vi "resonant.z.stack.run_rrMD.vi"() -> ()   [LabVIEW 2012]
doc: "SciScan 1.2 160622"
uses:
  Custom Controls/experiment type.ctl
  <vilib>/Utility/VariantDataType/Type.ctl
  GFG/GFGnumericGet.vi
  GFG/GFGfpRefGet.vi
  GFG/GFGbooleanGet.vi
  GFG/GFG library.lvlib
  <vilib>/Utility/VariantDataType/VariantType.lvlib
panel:
  out "error out 2":errorcluster
  out "transposed array":dbl[][](array[numeric])
  out "data":dbl[][](array[numeric])
  in  "error in (no error)":errorcluster
  out "error out":errorcluster
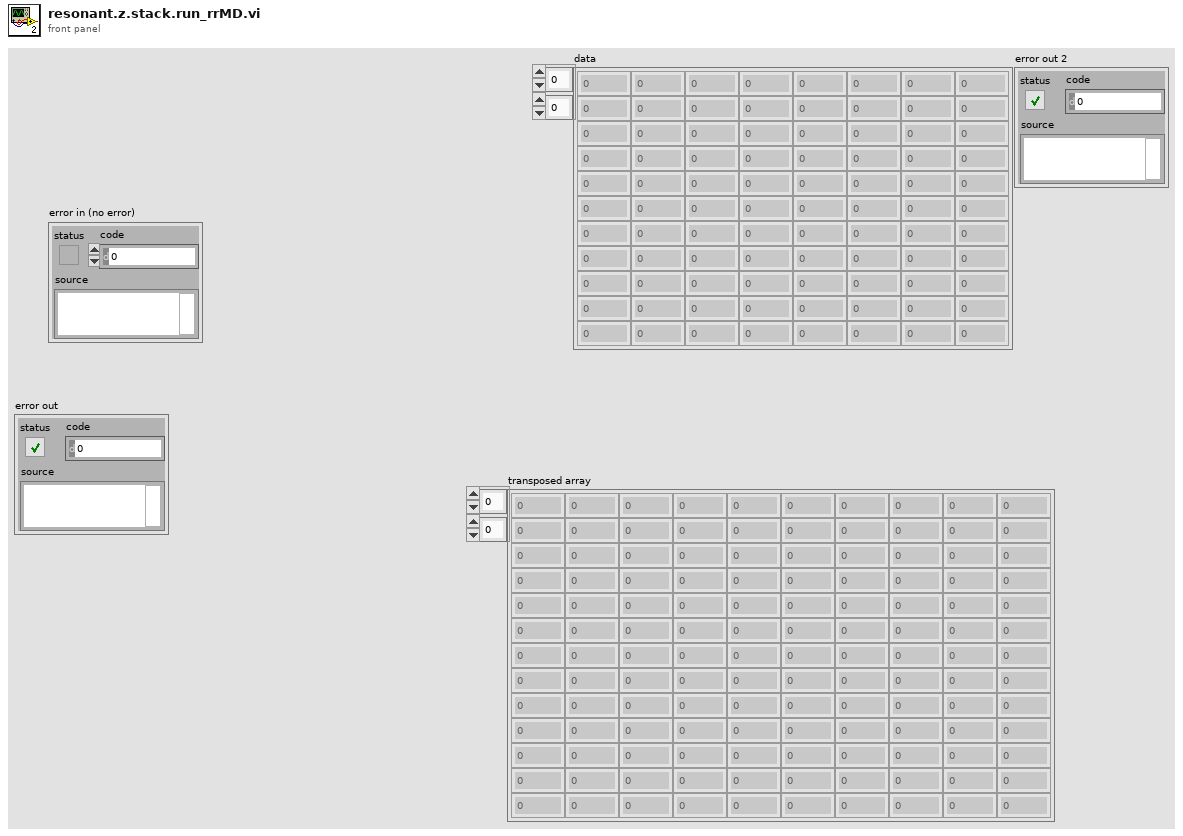
[diagram p1: front panel]
types:
  T1 = typedef "experiment type.ctl" = string
  T2 = enum8{"Enabled", "Disabled", "Disabled and Grayed Out"}
  T3 = cluster{"moveXabs":dbl, "moveYabs":dbl, "moveZabs":dbl}
  T4 = cluster{"WaveformChartRef":refnum<vi>, "DigitalRef":refnum<vi>, "ArrayRef":refnum<vi>, "TabControlRef":refnum<vi>, "EnumRef":refnum<vi>, "RingRef":refnum<vi>, "BooleanRef":refnum<vi>, "KnobRef":refnum<vi>, "SlideRef":refnum<vi>, "PathRef":refnum<vi>, "StringRef":refnum<vi>, "ComboBox":refnum<vi>, "WaveformGraphRef":refnum<vi>}
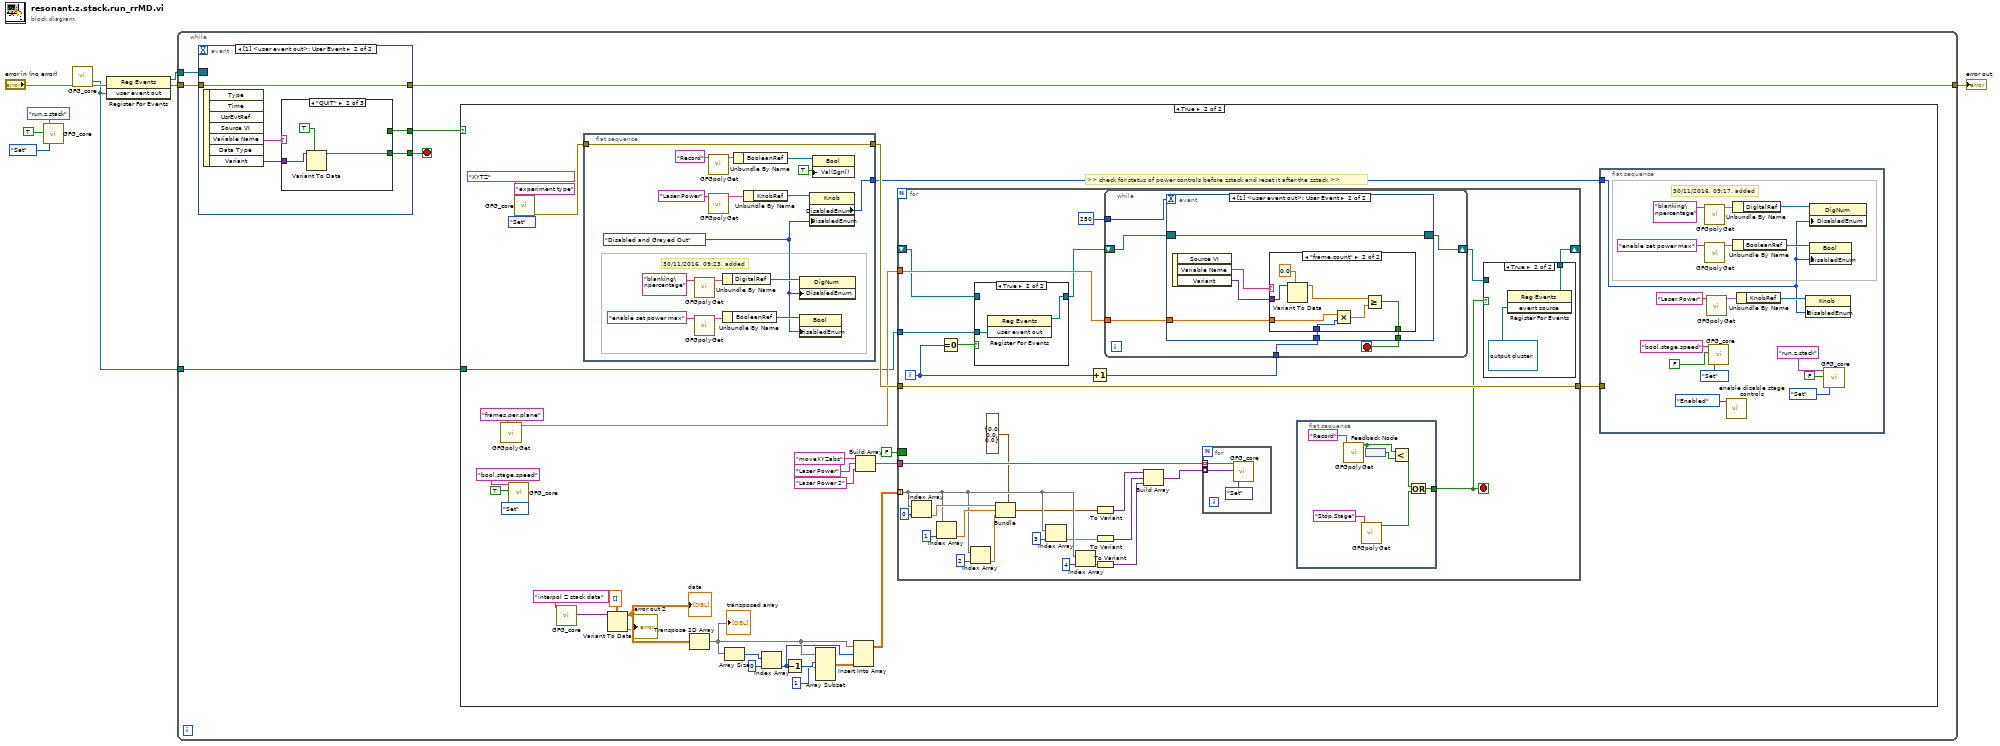
[diagram p0: block diagram]
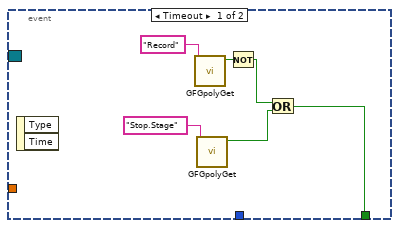
[diagram p5: hidden frame]
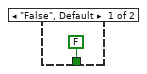
[diagram p6: hidden frame]
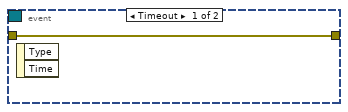
[diagram p7: hidden frame]
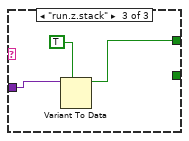
[diagram p9: hidden frame]
diagram:
  n1 = call "GFG_core.vi"("Variable Name in"="run.z.stack", "Variant in"=TRUE, "Action"=enum16{"Init", "Set", "Get"}."Set") -> ()  [unwired: 10 in, 7 out]
  n2 = call "GFG_core.vi"("error in (no error)"="error in (no error)") -> ("user event out"=w1:refnum<user-event>, "error out"=w6:errorcluster)  [unwired: 12 in, 5 out]
  n3 = register-events(error in=w6, w1) -> (reference out=w5:refnum<event-registration>, error out=w8:errorcluster)  [unwired: 1 in]
  n4 = while {
    tunnel: w5 -> [w15]
    tunnel: w8 -> [w14]
    tunnel: [w13] -> w9
    tunnel: w1 -> [w10]
    stop <- w12 stop-if-true
    n5 = event shown="[1] <user event out>: User Event" {
      selector: w15 -> [_ _]
      dyn-events: _ -> [_ _]
      timeout: _ -> [_ _]
      tunnel: w14 -> [w152 w157]
      tunnel: [w152 w157] -> w13
      tunnel: [_ w154] -> w12
      tunnel: [_ w153] -> w11
      event Timeout {
        n6 = event-data() -> ()  [unwired: 1 in, 2 out]
      }
      event User Event {
        n7 = event-data() -> ("Variable Name"=w156:string, "Variant"=w155:variant)  [unwired: 1 in, 5 out]
        n8 = case shown="\"QUIT\"" w156 {
          tunnel: w155 -> [_ w159 w162]
          tunnel: [_ w158 _] -> w154
          tunnel: [_ _ w161] -> w153
          frame "False", Default {
          }
          frame "QUIT" {
            n9 = Variant To Data(type=TRUE, Variant=w159) -> (data=w158:bool)  [unwired: 1 in, 1 out]
          }
          frame "run.z.stack" {
            n10 = Variant To Data(type=TRUE, Variant=w162) -> (data=w161:bool)  [unwired: 1 in, 1 out]
          }
        }
      }
    }
    n11 = case shown="True" w11 {
      tunnel: w10 -> [_ w17]
      frame False {
      }
      frame True {
        # ">> check for status of power controls before zstack and reset it after the zstack >>"
        n12 = call-poly "GFGpolyGet.vi"("Variable Name in"="frames.per.plane") -> ("Numeric"=w30:dbl)  [unwired: 8 in, 2 out]
        n13 = call "GFG_core.vi"("Variable Name in"="bool.stage.speed", "Variant in"=TRUE, "Action"=enum16{"Init", "Set", "Get"}."Set") -> ()  [unwired: 10 in, 7 out]
        n14 = call "GFG_core.vi"("Variable Name in"="experiment type", "Variant in"=T1 "XYTZ" ("experiment type"), "Action"=enum16{"Init", "Set", "Get"}."Set") -> ("error out"=w32:errorcluster)  [unwired: 10 in, 6 out]
        n15 = call "GFG_core.vi"("Variable Name in"="interpol Z stack data") -> ("Variant Out"=w44:variant)  [unwired: 12 in, 6 out]
        n16 = flat-sequence {
          tunnel: [w61] -> w33
          tunnel: w32 -> [w61]
          tunnel: [w47] -> w16
          frame #0 {
            w48 = T2."Disabled and Grayed Out" ("Disabled")
            # "30/11/2016, 09:23, added"
            n17 = call-poly "GFGpolyGet.vi"("Variable Name in"="blanking\npercentage") -> ("output cluster"=w53:T4)  [unwired: 9 in, 1 out]
            n18 = call-poly "GFGpolyGet.vi"("Variable Name in"="enable set power max") -> ("output cluster"=w50:T4)  [unwired: 9 in, 1 out]
            n19 = call-poly "GFGpolyGet.vi"("Variable Name in"="Record") -> ("output cluster"=w60:T4)  [unwired: 9 in, 1 out]
            n20 = call-poly "GFGpolyGet.vi"("Variable Name in"="Laser.Power") -> ("output cluster"=w55:T4)  [unwired: 9 in, 1 out]
            n21 = Unbundle By Name(w53) -> ("DigitalRef"=w54:refnum<vi>)
            n22 = Unbundle By Name(w50) -> ("BooleanRef"=w49:refnum<vi>)
            n23 = Unbundle By Name(w60) -> ("BooleanRef"=w59:refnum<vi>)
            n24 = Unbundle By Name(w55) -> ("KnobRef"=w57:refnum<vi>)
            n25 = property class="DigNum"(reference=w54, "DisabledEnum"=w48) -> ()  [unwired: 1 in, 2 out]
            n26 = property class="Bool"(reference=w49, "DisabledEnum"=w48) -> ()  [unwired: 1 in, 2 out]
            n27 = property class="Knob"(reference=w57, "DisabledEnum"=w48) -> ("DisabledEnum"=w47:T2)  [unwired: 1 in, 2 out]
            n28 = property class="Bool"(reference=w59, "Val(Sgnl)"=TRUE) -> ()  [unwired: 1 in, 2 out]
          }
        }
        n29 = Variant To Data(type=dbl[][] [] ("Interpolated Data"), Variant=w44) -> (data=w42:dbl[][], error out=→"error out 2":errorcluster)  [unwired: 1 in]
        "data" <- w42
        n30 = Transpose 2D Array(2D array=w42) -> (transposed array=w22:dbl[][])
        "transposed array" <- w22
        n31 = Array Size(array=w22) -> (size(s)=w26:i32[])
        n32 = Index Array(array=w26, index=0) -> (element=w20:i32)
        n33 = Decrement(x=w20) -> (x-1=w24:i32)
        n34 = Array Subset(array=w22, index (row)=w24, length (row)=1 ("length")) -> (w21:dbl[][])  [unwired: 2 in]
        n35 = Insert Into Array(array=w22, index (row)=w20, new element=w21) -> (w19:dbl[][])  [unwired: 1 in]
        n36 = Build Array("moveXYZabs" ("Variable Name in"), "Laser Power" ("Variable Name in"), "Laser Power 2" ("Variable Name in")) -> (w38:string[])
        n37 = for {
          tunnel: w19 -> [w100] mode=indexing
          tunnel: w38 -> [w109]
          tunnel: w33 -> [w90]
          tunnel: [w90] -> w34
          tunnel: w30 -> [w91]
          tunnel: w17 -> [w86]
          shift-right: [w82] -> _
          shift-left: _ -> [w84]
          border: FALSE ("Boolean Value OUT") -> [_]
          i -> [w88]
          stop <- w81 stop-if-true
          n38 = Index Array(array=w100, index=0) -> (element=w107:dbl)
          n39 = Index Array(array=w100, index=1) -> (element=w106:dbl)
          n40 = Equal To 0?(x=w88) -> (x = 0?=w87:bool)
          n41 = Index Array(array=w100, index=2) -> (element=w103:dbl)
          n42 = case shown="True" w87 {
            tunnel: w86 -> [_ w115]
            tunnel: [w113 w114] -> w85
            tunnel: w84 -> [w113 _]
            frame False {
            }
            frame True {
              n43 = register-events(w115) -> (reference out=w114:refnum<event-registration>)  [unwired: 2 in, 1 out]
            }
          }
          n44 = Bundle(cluster=T3 {"moveXabs"=0.0, "moveYabs"=0.0, "moveZabs"=0.0} ("output cluster"), "moveXabs"=w107, "moveYabs"=w106, "moveZabs"=w103) -> (w97:T3)
          n45 = Index Array(array=w100, index=3) -> (element=w98:dbl)
          n46 = Index Array(array=w100, index=4) -> (element=w99:dbl)
          n47 = Increment(x=w88) -> (x+1=w80:i32)
          n48 = To Variant(anything=w97) -> (Variant=w96:variant)
          n49 = To Variant(anything=w98) -> (Variant=w95:variant)
          n50 = To Variant(anything=w99) -> (Variant=w94:variant)
          n51 = while {
            tunnel: w91 -> [w120]
            tunnel: w80 -> [w119]
            tunnel: 250 -> [w117]
            shift-right: [w116] -> w83
            shift-left: w85 -> [w121]
            stop <- w118 stop-if-true
            n52 = event shown="[1] <user event out>: User Event" {
              selector: w121 -> [_ w128]
              dyn-events: [_ w128] -> w116
              timeout: w117 -> [_ _]
              tunnel: w120 -> [_ w131]
              tunnel: w119 -> [_ w130]
              tunnel: [w122 w129] -> w118
              event Timeout {
                n53 = event-data() -> ()  [unwired: 1 in, 2 out]
                n54 = call-poly "GFGpolyGet.vi"("Variable Name in"="Record") -> ("Boolean Value OUT"=w125:bool)  [unwired: 9 in, 1 out]
                n55 = call-poly "GFGpolyGet.vi"("Variable Name in"="Stop.Stage") -> ("Boolean Value OUT"=w126:bool)  [unwired: 9 in, 1 out]
                n56 = Not(x=w125) -> (.not. x?=w127:bool)
                n57 = Or(x=w127, y=w126) -> (x .or. y?=w122:bool)
              }
              event User Event {
                n58 = event-data() -> ("Variable Name"=w133:string, "Variant"=w132:variant)  [unwired: 1 in, 1 out]
                n59 = case shown="\"frame.count\"" w133 {
                  tunnel: w132 -> [_ w141]
                  tunnel: w131 -> [_ w139]
                  tunnel: w130 -> [_ w138]
                  tunnel: [FALSE w135] -> w129
                  frame "False", Default {
                  }
                  frame "frame.count" {
                    n60 = Variant To Data(type=0.0, Variant=w141) -> (data=w136:dbl)  [unwired: 1 in, 1 out]
                    n61 = Multiply(x=w139, y=w138) -> (x*y=w137:dbl)
                    n62 = Greater Or Equal?(x=w136, y=w137) -> (x >= y?=w135:bool)
                  }
                }
              }
            }
          }
          n63 = Build Array(w96, w95, w94) -> (w93:variant[])
          n64 = for {
            tunnel: w93 -> [w150] mode=indexing
            tunnel: w109 -> [w151] mode=indexing
            n65 = call "GFG_core.vi"("Variable Name in"=w151, "Variant in"=w150, "Action"=enum16{"Init", "Set", "Get"}."Set") -> ()  [unwired: 10 in, 7 out]
          }
          n66 = flat-sequence {
            tunnel: [w146] -> w81
            frame #0 {
              n67 = call-poly "GFGpolyGet.vi"("Variable Name in"="Record") -> ("Boolean Value OUT"=w145:bool)  [unwired: 9 in, 1 out]
              n68 = call-poly "GFGpolyGet.vi"("Variable Name in"="Stop.Stage") -> ("Boolean Value OUT"=w144:bool)  [unwired: 9 in, 1 out]
              n69 = feedback-in #1(w145) -> ()
              n70 = feedback #1() -> (w142:bool)
              n71 = Less?(x=w145, y=w142) -> (x < y?=w143:bool)
              n72 = Or(x=w143, y=w144) -> (x .or. y?=w146:bool)
            }
          }
          n73 = case shown="True" w81 {
            tunnel: [w110 w112] -> w82
            tunnel: w83 -> [w110 _]
            frame False {
            }
            frame True {
              n74 = register-events(refnum<user-event> refnum ("event source")) -> (reference out=w112:refnum<event-registration>)  [unwired: 2 in, 1 out]
            }
          }
        }
        n75 = flat-sequence {
          tunnel: w34 -> [_]
          tunnel: w16 -> [w63]
          frame #0 {
            # "30/11/2016, 09:17, added"
            n76 = call-poly "GFGpolyGet.vi"("Variable Name in"="blanking\npercentage") -> ("output cluster"=w68:T4)  [unwired: 9 in, 1 out]
            n77 = call-poly "GFGpolyGet.vi"("Variable Name in"="enable set power max") -> ("output cluster"=w65:T4)  [unwired: 9 in, 1 out]
            n78 = call-poly "GFGpolyGet.vi"("Variable Name in"="Laser.Power") -> ("output cluster"=w70:T4)  [unwired: 9 in, 1 out]
            n79 = call "GFG_core.vi"("Variable Name in"="bool.stage.speed", "Variant in"=FALSE, "Action"=enum16{"Init", "Set", "Get"}."Set") -> ()  [unwired: 10 in, 7 out]
            n80 = call "enable disable stage controls.vi"("Disabled"=T2."Enabled") -> ()  [unwired: 11 in]
            n81 = Unbundle By Name(w68) -> ("DigitalRef"=w69:refnum<vi>)
            n82 = Unbundle By Name(w65) -> ("BooleanRef"=w64:refnum<vi>)
            n83 = Unbundle By Name(w70) -> ("KnobRef"=w72:refnum<vi>)
            n84 = property class="Knob"(reference=w72, "DisabledEnum"=w63) -> ()  [unwired: 1 in, 2 out]
            n85 = property class="DigNum"(reference=w69, "DisabledEnum"=w63) -> ()  [unwired: 1 in, 2 out]
            n86 = property class="Bool"(reference=w64, "DisabledEnum"=w63) -> ()  [unwired: 1 in, 2 out]
            n87 = call "GFG_core.vi"("Variable Name in"="run.z.stack", "Variant in"=FALSE, "Action"=enum16{"Init", "Set", "Get"}."Set") -> ()  [unwired: 10 in, 7 out]
          }
        }
      }
    }
  }
  "error out" <- w9
